vi "EnglishTeacherSM_main.vi"() -> ()   [LabVIEW 2020]
uses:
  #typedef_English_Teacher_States.ctl
  #typedef_WordsActions.ctl
panel:
  in  "Test":bool
  in  "Learining":bool
  in  "Exit":bool
  in  "Stop":bool
  in  "Angielski":string
  in  "Polski":string
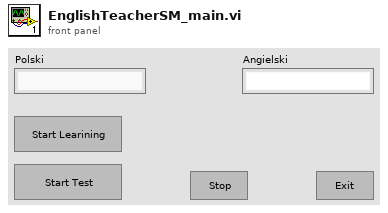
[diagram p1: front panel]
types:
  T1 = typedef "#typedef_English_Teacher_States.ctl" = enum16{"Initialize", "Idle", "Learning_1", "Learning_2", "Learning_3", "Test_1", "Test_2", "Test_3", "Test_4", "Stop", "Exit"}
  T2 = typedef "#typedef_WordsActions.ctl" = enum16{"ShowPolish", "ShowEnglish", "ShowBoth", "ShowNone"}
  T3 = enum8{"Enabled", "Disabled", "Disabled and Grayed Out"}
  T4 = typedef "#typedef_Program_Data.ctl" = cluster{"WaitTime":dbl, "PolishWords":string[], "EnglishWords":string[], "PairNumbers":i32, "NextState":T1, "WordsAction":T2, "CurrentPairNum":i32, "CurrentEnglishWord":string}
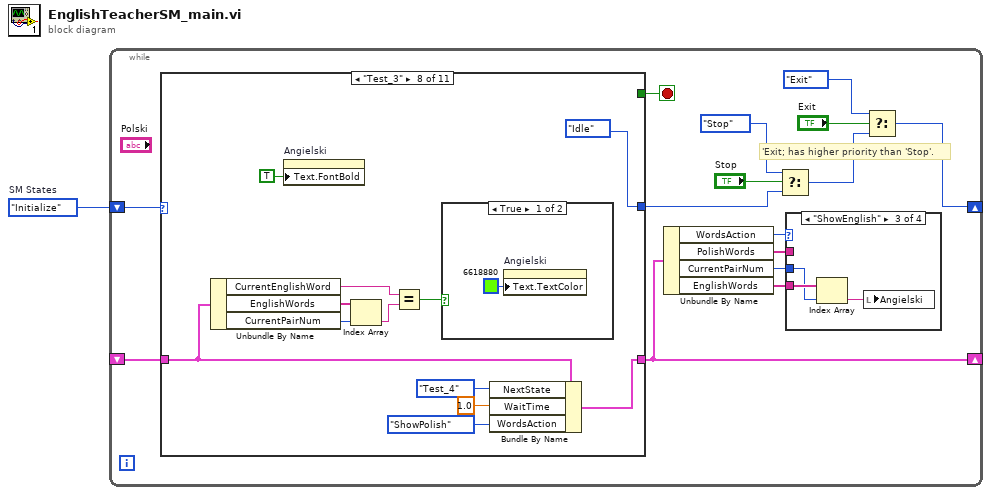
[diagram p0: block diagram]
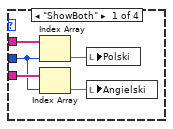
[diagram p2: hidden frame]
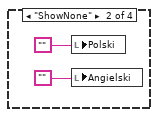
[diagram p3: hidden frame]
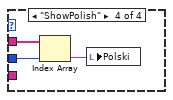
[diagram p4: hidden frame]
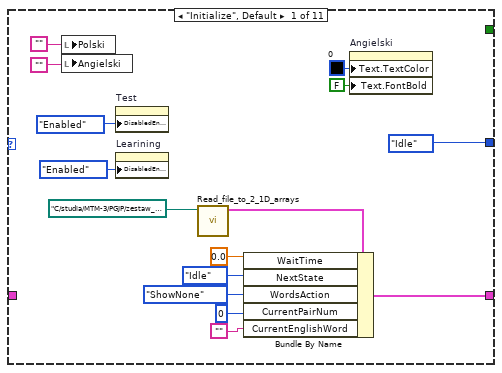
[diagram p5: hidden frame]
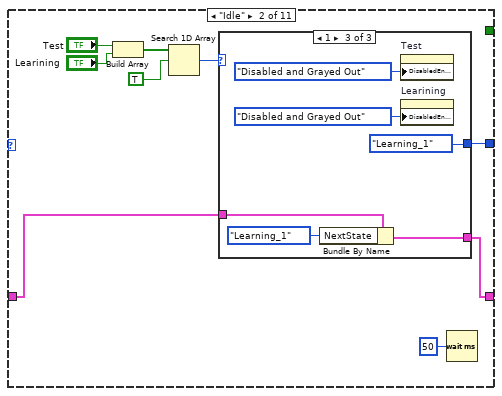
[diagram p6: hidden frame]
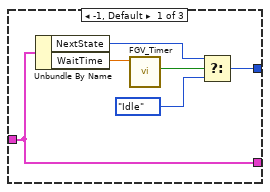
[diagram p7: hidden frame]
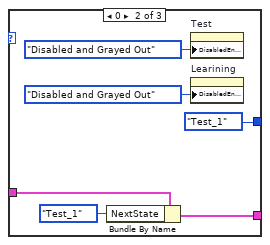
[diagram p8: hidden frame]
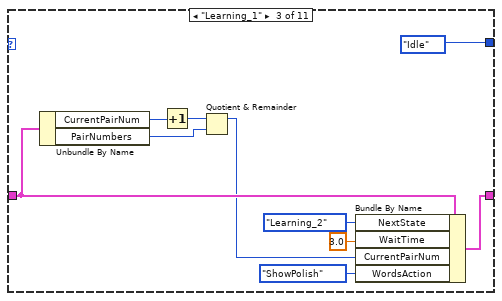
[diagram p9: hidden frame]
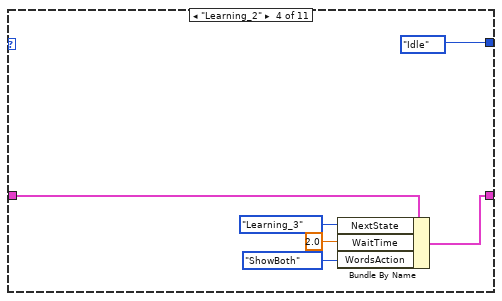
[diagram p10: hidden frame]
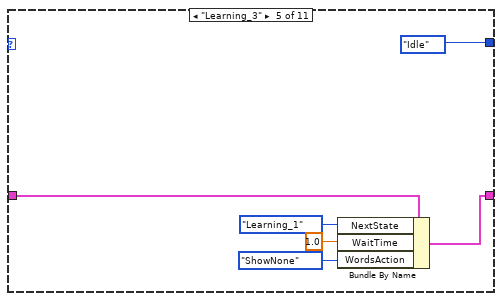
[diagram p11: hidden frame]
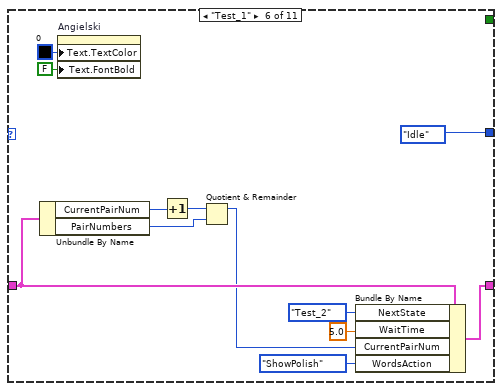
[diagram p12: hidden frame]
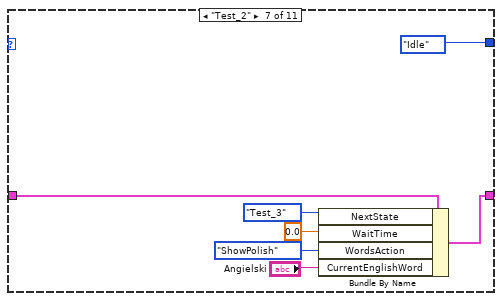
[diagram p13: hidden frame]
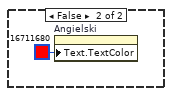
[diagram p14: hidden frame]
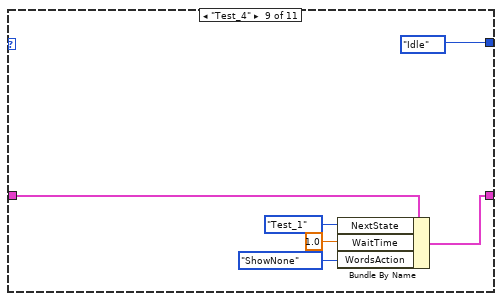
[diagram p15: hidden frame]
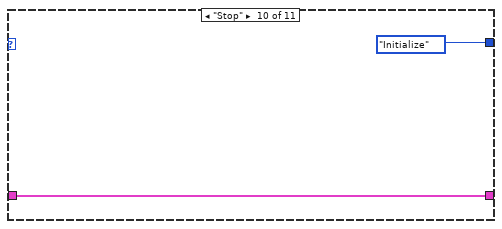
[diagram p16: hidden frame]
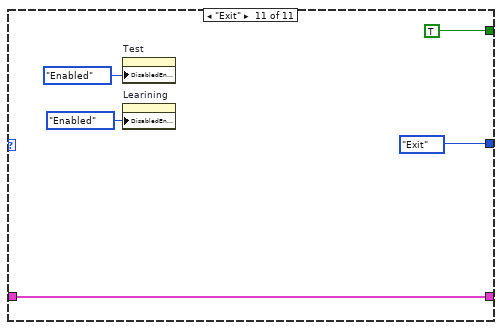
[diagram p17: hidden frame]
diagram:
  w1 = #typedef_English_Teacher_States."Initialize"  # SM States
  n1 = while {
    shift-right: [w11] -> _
    shift-left: w1 -> [w10]
    shift-right: [w2] -> _
    shift-left: _ -> [w7]
    stop <- w8 stop-if-true
    # "'Exit; has higher priority than 'Stop'."
    n2 = case shown="\"Test_3\"" w10 {
      tunnel: [#typedef_English_Teacher_States."Idle" ("SM States") w49 #typedef_English_Teacher_States."Idle" ("SM States") #typedef_English_Teacher_States."Idle" ("SM States") #typedef_English_Teacher_States."Idle" ("SM States") #typedef_English_Teacher_States."Idle" ("SM States") #typedef_English_Teacher_States."Idle" ("SM States") #typedef_English_Teacher_States."Idle" ("SM States") #typedef_English_Teacher_States."Idle" ("SM States") #typedef_English_Teacher_States."Initialize" ("SM States") #typedef_English_Teacher_States."Exit" ("SM States")] -> w9
      tunnel: [_ _ _ _ _ _ _ _ _ _ TRUE] -> w8
      tunnel: w7 -> [_ w47 w77 w86 w92 w101 w111 w119 w131 w133 w137]
      tunnel: [w39 w46 w80 w85 w91 w104 w110 w123 w130 w133 w137] -> w2
      frame "Initialize", Default {
        n3 = local write "Polski"("") -> ()
        n4 = local write "Angielski"("") -> ()
        n5 = property on="Test" class="Bool"("DisabledEnum"=T3."Enabled" ("Disabled")) -> ()  [unwired: 2 in, 2 out]
        n6 = property on="Learining" class="Bool"("DisabledEnum"=T3."Enabled" ("Disabled")) -> ()  [unwired: 2 in, 2 out]
        n7 = call "Read_file_to_2_1D_arrays.vi"("Path"=path "C:/studia/MTM-3/PGJP/zestaw_8/EnglishTeacher_SM/dictionary.txt") -> ("ProgramData"=w36:T4)  [unwired: 9 in, 1 out]
        n8 = Bundle By Name(cluster=w36, "WaitTime"=0.0, "NextState"=#typedef_English_Teacher_States."Idle", "WordsAction"=#typedef_WordsActions."ShowNone", "CurrentPairNum"=0 ("CurrentPairNumber"), "CurrentEnglishWord"="") -> (w39:T4)
        n9 = property on="Angielski" class="Str"("Text.TextColor"=u32 0 ("Text.Text Colors:BG Color"), "Text.FontBold"=FALSE ("Text.Font:Bold")) -> ()  [unwired: 2 in, 2 out]
      }
      frame "Idle" {
        n10 = Build Array("Test", "Learining") -> (w52:bool[])
        n11 = Search 1D Array(1D array=w52, element=TRUE) -> (index of element=w48:i32)  [unwired: 1 in]
        n12 = case shown="1" w48 {
          tunnel: [w56 #typedef_English_Teacher_States."Test_1" ("SM States") #typedef_English_Teacher_States."Learning_1" ("SM States")] -> w49
          tunnel: w47 -> [w59 w62 w68]
          tunnel: [w59 w61 w67] -> w46
          frame -1, Default {
            n13 = Unbundle By Name(w59) -> ("NextState"=w57:T1, "WaitTime"=w54:dbl)
            n14 = call "FGV_Timer.vi"("TimeToElapse (10) (s)"=w54) -> ("Time Elapsed?"=w58:bool)  [unwired: 8 in, 2 out]
            n15 = Select(t=w57, s=w58, f=#typedef_English_Teacher_States."Idle") -> (s? t:f=w56:T1)
          }
          frame 0 {
            n16 = Bundle By Name(cluster=w62, "NextState"=#typedef_English_Teacher_States."Test_1") -> (w61:T4)
            n17 = property on="Test" class="Bool"("DisabledEnum"=T3."Disabled and Grayed Out" ("Disabled")) -> ()  [unwired: 2 in, 2 out]
            n18 = property on="Learining" class="Bool"("DisabledEnum"=T3."Disabled and Grayed Out" ("Disabled")) -> ()  [unwired: 2 in, 2 out]
          }
          frame 1 {
            n19 = Bundle By Name(cluster=w68, "NextState"=#typedef_English_Teacher_States."Learning_1") -> (w67:T4)
            n20 = property on="Test" class="Bool"("DisabledEnum"=T3."Disabled and Grayed Out" ("Disabled")) -> ()  [unwired: 2 in, 2 out]
            n21 = property on="Learining" class="Bool"("DisabledEnum"=T3."Disabled and Grayed Out" ("Disabled")) -> ()  [unwired: 2 in, 2 out]
          }
        }
        n22 = Wait (ms)(milliseconds to wait=u32 50) -> ()  [unwired: 1 out]
      }
      frame "Learning_1" {
        n23 = Unbundle By Name(w77) -> ("CurrentPairNum"=w76:i32, "PairNumbers"=w74:i32)
        n24 = Increment(x=w76) -> (x+1=w75:i32)
        n25 = Quotient & Remainder(x=w75, y=w74) -> (x-y*floor(x/y)=w73:i32)  [unwired: 1 out]
        n26 = Bundle By Name(cluster=w77, "NextState"=#typedef_English_Teacher_States."Learning_2", "WaitTime"=3.0, "CurrentPairNum"=w73, "WordsAction"=#typedef_WordsActions."ShowPolish") -> (w80:T4)
      }
      frame "Learning_2" {
        n27 = Bundle By Name(cluster=w86, "NextState"=#typedef_English_Teacher_States."Learning_3", "WaitTime"=2.0, "WordsAction"=#typedef_WordsActions."ShowBoth") -> (w85:T4)
      }
      frame "Learning_3" {
        n28 = Bundle By Name(cluster=w92, "NextState"=#typedef_English_Teacher_States."Learning_1", "WaitTime"=1.0, "WordsAction"=#typedef_WordsActions."ShowNone") -> (w91:T4)
      }
      frame "Test_1" {
        n29 = Unbundle By Name(w101) -> ("CurrentPairNum"=w100:i32, "PairNumbers"=w98:i32)
        n30 = property on="Angielski" class="Str"("Text.TextColor"=u32 0 ("Text.Text Colors:BG Color"), "Text.FontBold"=FALSE ("Text.Font:Bold")) -> ()  [unwired: 2 in, 2 out]
        n31 = Increment(x=w100) -> (x+1=w99:i32)
        n32 = Quotient & Remainder(x=w99, y=w98) -> (x-y*floor(x/y)=w97:i32)  [unwired: 1 out]
        n33 = Bundle By Name(cluster=w101, "NextState"=#typedef_English_Teacher_States."Test_2", "WaitTime"=5.0, "CurrentPairNum"=w97, "WordsAction"=#typedef_WordsActions."ShowPolish") -> (w104:T4)
      }
      frame "Test_2" {
        n34 = Bundle By Name(cluster=w111, "NextState"=#typedef_English_Teacher_States."Test_3", "WaitTime"=0.0, "WordsAction"=#typedef_WordsActions."ShowPolish", "CurrentEnglishWord"="Angielski") -> (w110:T4)
      }
      frame "Test_3" {
        n35 = Unbundle By Name(w119) -> ("CurrentEnglishWord"=w113:string, "EnglishWords"=w118:string[], "CurrentPairNum"=w117:i32)
        n36 = property on="Angielski" class="Str"("Text.FontBold"=TRUE ("Text.Font:Bold")) -> ()  [unwired: 2 in, 2 out]
        n37 = Index Array(array=w118, index=w117) -> (element=w116:string)
        n38 = Equal?(x=w113, y=w116) -> (x = y?=w115:bool)
        n39 = case shown="True" w115 {
          frame True {
            n40 = property on="Angielski" class="Str"("Text.TextColor"=u32 6618880 ("Text.Text Colors:BG Color")) -> ()  [unwired: 2 in, 2 out]
          }
          frame False {
            n41 = property on="Angielski" class="Str"("Text.TextColor"=u32 16711680 ("Text.Text Colors:BG Color")) -> ()  [unwired: 2 in, 2 out]
          }
        }
        n42 = Bundle By Name(cluster=w119, "NextState"=#typedef_English_Teacher_States."Test_4", "WaitTime"=1.0, "WordsAction"=#typedef_WordsActions."ShowPolish") -> (w123:T4)
      }
      frame "Test_4" {
        n43 = Bundle By Name(cluster=w131, "NextState"=#typedef_English_Teacher_States."Test_1", "WaitTime"=1.0, "WordsAction"=#typedef_WordsActions."ShowNone") -> (w130:T4)
      }
      frame "Stop" {
      }
      frame "Exit" {
        n44 = property on="Test" class="Bool"("DisabledEnum"=T3."Enabled" ("Disabled")) -> ()  [unwired: 2 in, 2 out]
        n45 = property on="Learining" class="Bool"("DisabledEnum"=T3."Enabled" ("Disabled")) -> ()  [unwired: 2 in, 2 out]
      }
    }
    n46 = Unbundle By Name(w2) -> ("WordsAction"=w6:T2, "PolishWords"=w5:string[], "CurrentPairNum"=w4:i32, "EnglishWords"=w3:string[])
    n47 = Select(t=#typedef_English_Teacher_States."Stop" ("SM States"), s="Stop", f=w9) -> (s? t:f=w13:T1)
    n48 = case shown="\"ShowEnglish\"" w6 {
      tunnel: w5 -> [w21 _ _ w29]
      tunnel: w4 -> [w19 _ w25 w28]
      tunnel: w3 -> [w20 _ w26 _]
      frame "ShowBoth" {
        n49 = Index Array(array=w21, index=w19) -> (element=w18:string)
        n50 = Index Array(array=w20, index=w19) -> (element=w17:string)
        n51 = local write "Polski"(w18) -> ()
        n52 = local write "Angielski"(w17) -> ()
      }
      frame "ShowNone" {
        n53 = local write "Polski"("") -> ()
        n54 = local write "Angielski"("") -> ()
      }
      frame "ShowEnglish" {
        n55 = Index Array(array=w26, index=w25) -> (element=w24:string)
        n56 = local write "Angielski"(w24) -> ()
      }
      frame "ShowPolish" {
        n57 = Index Array(array=w29, index=w28) -> (element=w27:string)
        n58 = local write "Polski"(w27) -> ()
      }
    }
    n59 = Select(t=#typedef_English_Teacher_States."Exit", s="Exit", f=w13) -> (s? t:f=w11:T1)
  }
